vi "Record Queue Commands.vi"(8 "error in (no error)":errorcluster, 11 "queue In":refnum<queue>) -> (0 "error out":errorcluster, 1 "Record command count":i32, 2 "Record File Path":path, 3 "queue Out":refnum<queue>)   [LabVIEW 2016]
uses:
  <vilib>/NI Veristand/Display Template Support/Display Template Support.llb/enum_Graph Handler Message.ctl
  <vilib>/NI Veristand/Display Template Support/Display Template Support.llb/cluster_Graph Handler Message.ctl
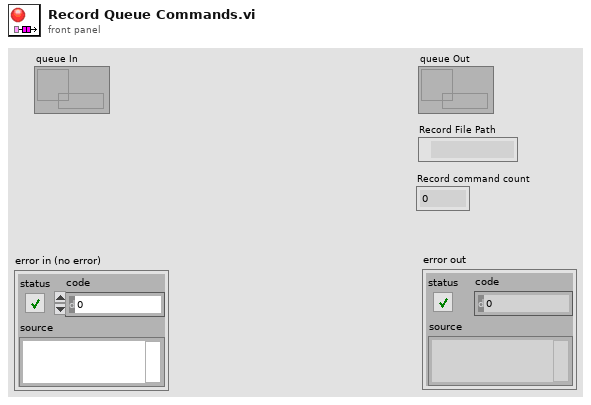
[diagram p1: front panel]
types:
  T1 = typedef "cluster_Graph Handler Message.ctl" = cluster{"Message":T2, "Data":variant}
  T2 = typedef "enum_Graph Handler Message.ctl" = enum16{"None", "Stop", "Hold", "Update Channels", "New Settings", "Control Value", "Edit Value"}
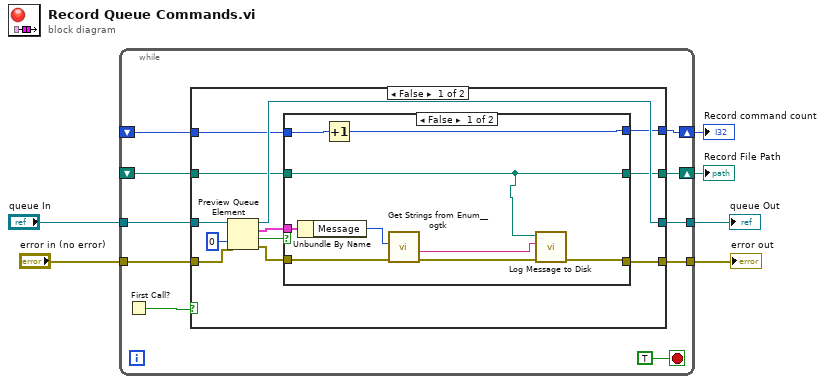
[diagram p0: block diagram]
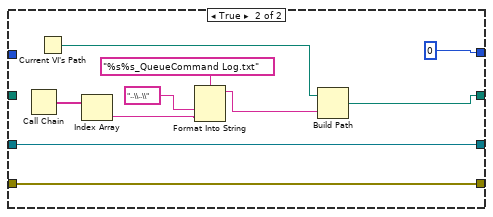
[diagram p3: hidden frame]
diagram:
  n1 = while {
    tunnel: "queue In" -> [w14]
    tunnel: [w13] -> w5
    tunnel: [w12] -> w4
    tunnel: "error in (no error)" -> [w11]
    shift-right: [w9] -> w1
    shift-left: _ -> [w8]
    shift-right: [w10] -> w2
    shift-left: _ -> [w7]
    stop <- TRUE stop-if-true
    n2 = First Call?() -> (First Call?: T/F=w16:bool)
    n3 = case shown="False" w16 {
      tunnel: w14 -> [w28 w50]
      tunnel: [w22 w50] -> w13
      tunnel: [w24 w49] -> w12
      tunnel: w11 -> [w27 w49]
      tunnel: [w20 w47] -> w10
      tunnel: [w19 0] -> w9
      tunnel: w8 -> [w18 _]
      tunnel: w7 -> [w17 _]
      frame False {
        n4 = Preview Queue Element(queue=w28, timeout in ms (-1)=0, error in (no error)=w27) -> (queue out=w22:refnum<queue>, element=w21:T1, timed out?=w25:bool, error out=w23:errorcluster)
        n5 = case shown="False" w25 {
          tunnel: [w32 w40] -> w24
          tunnel: w23 -> [w35 w40]
          tunnel: w21 -> [w37 _]
          tunnel: [w31 w38] -> w20
          tunnel: [w29 w39] -> w19
          tunnel: w18 -> [w30 w39]
          tunnel: w17 -> [w31 w38]
          frame False {
            n6 = Unbundle By Name(w37) -> ("Message"=w36:T2)
            n7 = Increment(x=w30) -> (x+1=w29:i32)
            n8 = call <userlib>:"Get Strings from Enum__ogtk.vi"("error in (no error)"=w35, "Enum"=w36) -> ("error out"=w34:errorcluster, "String Value"=w33:string)  [unwired: 6 in, 2 out]
            n9 = call <userlib>:"Log Message to Disk.vi"("error in (no error)"=w34, "Message"=w33, "Log File Path (FM_debug.txt)"=w31) -> ("error out"=w32:errorcluster)  [unwired: 8 in]
          }
          frame True {
          }
        }
      }
      frame True {
        n10 = Call Chain() -> (call chain=w44:string[])
        n11 = Current VI's Path() -> (path=w46:path)
        n12 = Index Array(array=w44) -> (element=w42:string)  [unwired: 1 in]
        n13 = Format Into String(format string="%s%s_QueueCommand Log.txt", "..\\..\\" ("input 1"), w42) -> (resulting string=w43:string)  [unwired: 2 in, 1 out]
        n14 = Build Path(base path=w46, name or relative path=w43) -> (appended path=w47:path)
      }
    }
  }
  "queue Out" <- w5
  "error out" <- w4
  "Record File Path" <- w2
  "Record command count" <- w1
